vi "Logging Message Loop.vi"(8 "error in (no error)":errorcluster, 10 "Data Queue":refnum<queue>, 11 "Message Queues":T1) -> (0 "error out":errorcluster)   [LabVIEW 2017, in "Logging.lvlib"]
doc: "The message loop subVI to handle messages pertaining to logging data."
uses:
  Logging.lvlib
  support/Message Queue/All Message Queues.ctl
  support/Message Queue/Message Cluster.ctl
  Logging Configuration.ctl
  Logging State.ctl
  support/Message Queue/Enqueue Message (Single).vi
  <vilib>/Utility/error.llb/Error Cluster From Error Code.vi
  <vilib>/ErrorRing/Error Ring.xnode
  support/Message Queue/Message Queue.lvlib
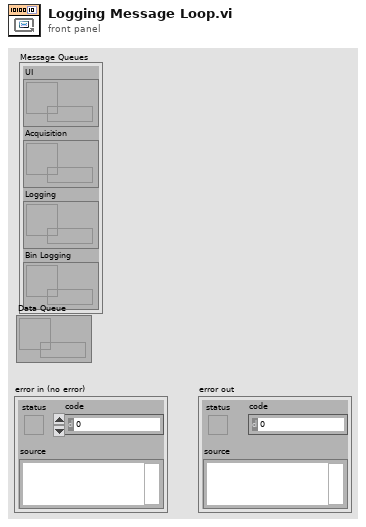
[diagram p1: front panel]
types:
  T1 = typedef "Message Queue.lvlib/All Message Queues.ctl" = cluster{"UI":refnum<queue>, "Acquisition":refnum<queue>, "Logging":refnum<queue>, "Bin Logging":refnum<queue>}
  T2 = typedef "Logging.lvlib/Logging Configuration.ctl" = cluster{"Log File Base Path":path, "TDMS File Reference":refnum<k34>, "Log File Offsite Path":path, "Offsite storage?":bool, "Project code":string, "Max writing time to a file [min]":dbl, "Bin File Reference":refnum<file>}
  T3 = typedef "Logging.lvlib/Logging State.ctl" = enum16{"Idle", "Logging"}
  T4 = enum16{"open", "open or create", "create or replace", "create", "open (read-only)"}
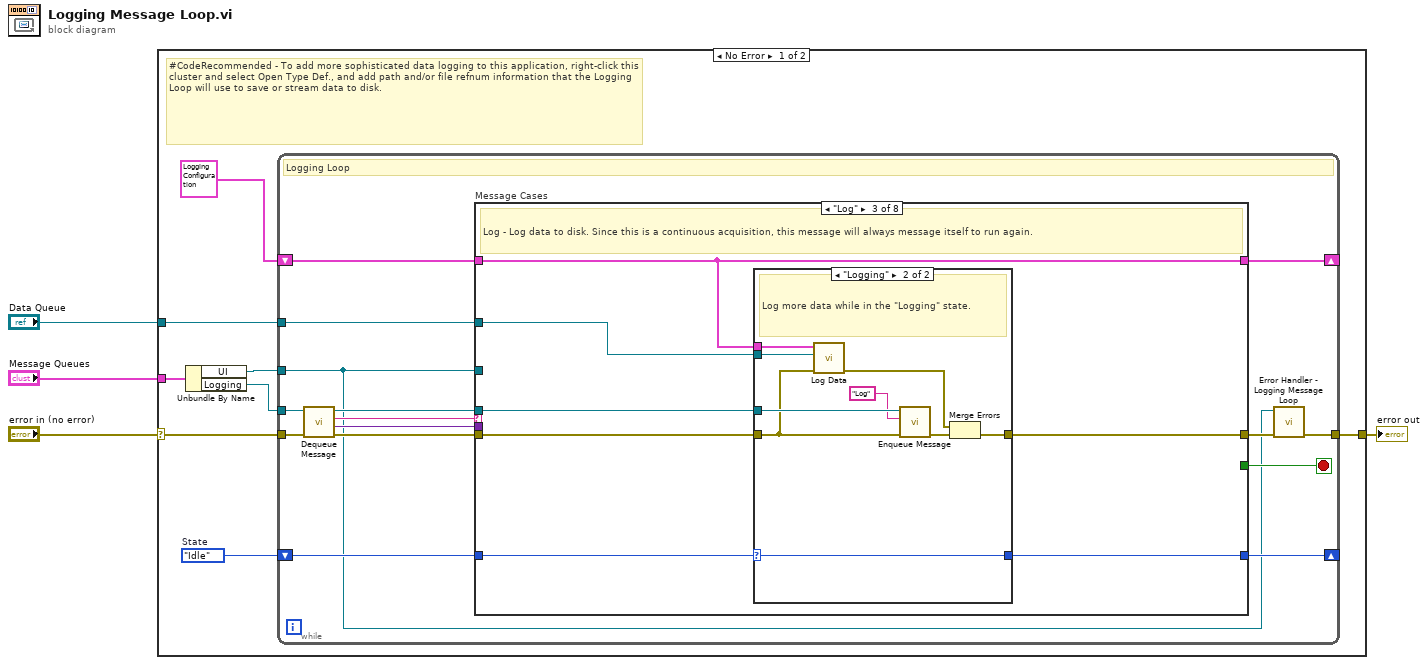
[diagram p0: block diagram]
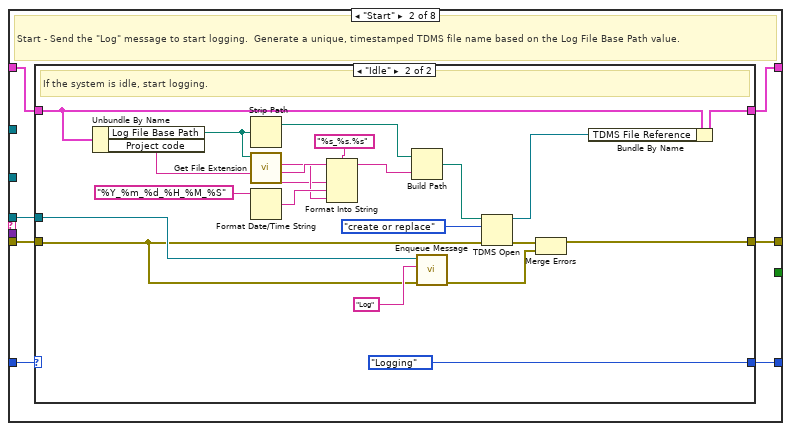
[diagram p3: hidden frame]
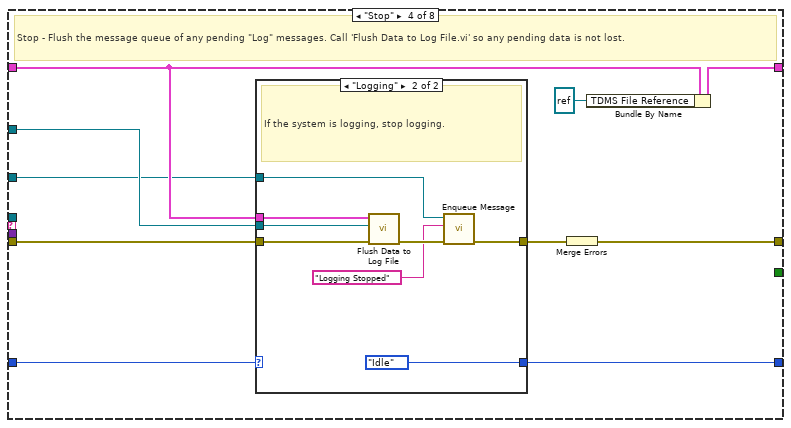
[diagram p6: hidden frame]
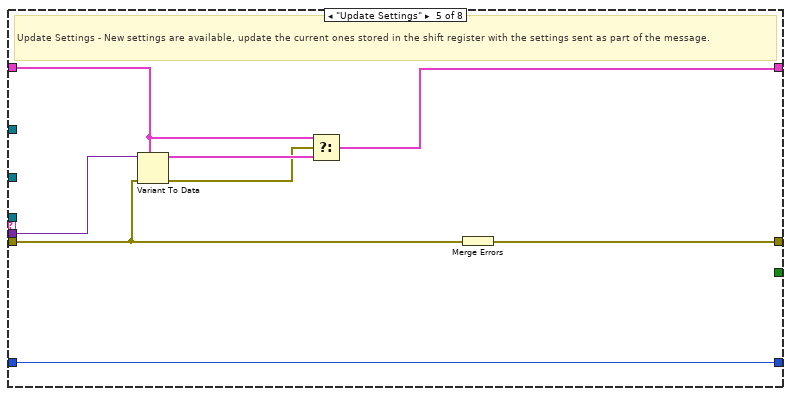
[diagram p8: hidden frame]
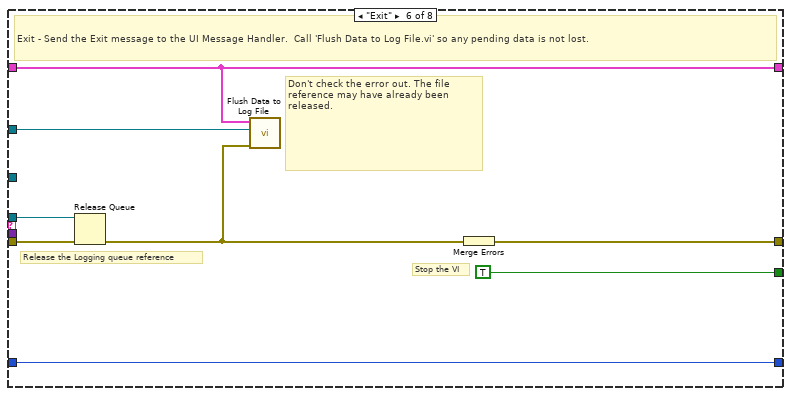
[diagram p9: hidden frame]
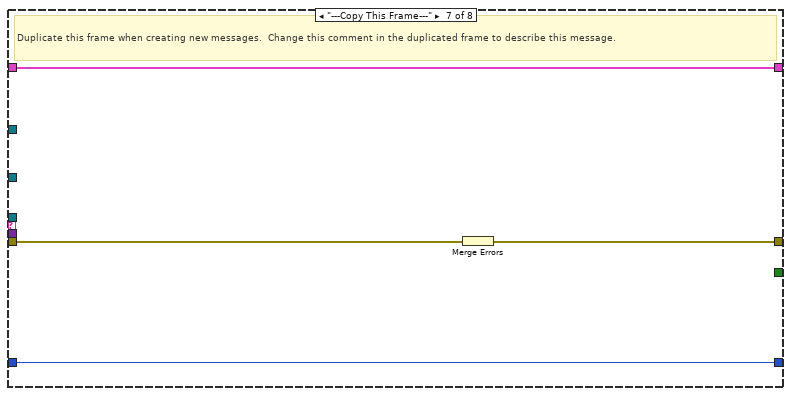
[diagram p10: hidden frame]
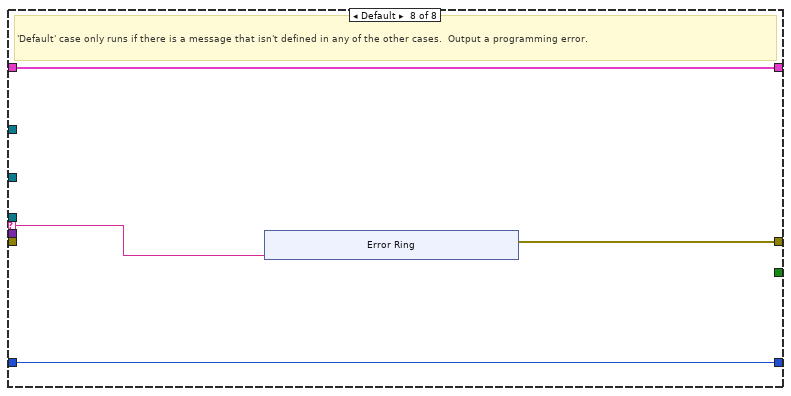
[diagram p11: hidden frame]
diagram:
  n1 = case shown="No Error" "error in (no error)" {
    selector: "error in (no error)" -> [w8 w131]
    tunnel: "Message Queues" -> [w12 _]
    tunnel: [w10 w131] -> w3
    tunnel: "Data Queue" -> [w7 _]
    frame No Error {
      w5 = Logging_State."Idle"  # State
      # "#CodeRecommended - To add more sophisticated data logging to this application, right-click this cluster and select Open Type Def., and add path and/or file refnum information that the Logging Loop will use to save or stream data to disk."
      n2 = Unbundle By Name(w12) -> ("UI"=w6:refnum<queue>, "Logging"=w11:refnum<queue>)
      n3 = while {
        tunnel: w11 -> [w19]
        shift-right: [w26] -> _
        shift-left: T2 {"Log File Base Path"=path "", "TDMS File Reference"=refnum, "Log File Offsite Path"=path "", "Offsite storage?"=FALSE, "Project code"="", "Max writing time to a file [min]"=0.0, "Bin File Reference"=refnum} ("Logging Configuration") -> [w27]
        tunnel: w6 -> [w13]
        tunnel: w7 -> [w18]
        shift-right: [w16] -> _
        shift-left: w5 -> [w17]
        tunnel: w8 -> [w24]
        tunnel: [w15] -> w10
        stop <- w25 stop-if-true
        # "Logging Loop"
        n4 = call "Dequeue Message.vi"("error in (no error)"=w24, "Message Queue"=w19) -> ("error out"=w23:errorcluster, "Message Data"=w21:variant, "Message"=w22:string, "dup Message Queue"=w20:refnum<queue>)  [unwired: 6 in]
        n5 = case "Message Cases" shown="\"Log\"" w22 {
          selector: w22 -> [_ _ _ _ _ _ _ w120]
          tunnel: w20 -> [_ w36 w67 _ _ w112 _ _]
          tunnel: w23 -> [w29 w35 w65 w83 w101 w113 w119 _]
          tunnel: [w29 w37 w68 w89 w107 w114 w117 w121] -> w14
          tunnel: w27 -> [w30 w34 w64 w84 w105 w110 w118 w123]
          tunnel: [w30 w33 w64 w87 w102 w110 w118 w123] -> w26
          tunnel: [_ _ _ _ _ TRUE _ _] -> w25
          tunnel: w21 -> [_ _ _ _ w106 _ _ _]
          tunnel: w13 -> [_ _ _ w80 _ _ _ _]
          tunnel: w18 -> [_ _ w66 w85 _ w109 _ _]
          tunnel: w17 -> [w28 w32 w63 w82 w100 w108 w116 w122]
          tunnel: [w28 w31 w62 w81 w100 w108 w116 w122] -> w16
          frame "Initialize" {
            # "Initialize - gets called when first launched. Currently a no-op."
          }
          frame "Start" {
            # "Start - Send the \"Log\" message to start logging.  Generate a unique, timestamped TDMS file name based on the Log File Base Path value."
            n6 = case shown="\"Idle\"" w32 {
              selector: w32 -> [w39 _]
              tunnel: [w38 w43] -> w37
              tunnel: w36 -> [_ w44]
              tunnel: w35 -> [w38 w42]
              tunnel: w34 -> [w40 w45]
              tunnel: [w40 w47] -> w33
              tunnel: [w39 Logging_State."Logging" ("State")] -> w31
              frame "Logging" {
                # "The system is already logging. Ignore the \"Start\" message."
              }
              frame "Idle" {
                # "If the system is idle, start logging."
                n7 = Unbundle By Name(w45) -> ("Log File Base Path"=w60:path, "Project code"=w41:string)
                n8 = Strip Path(path=w60) -> (stripped path=w57:path)  [unwired: 1 out]
                n9 = call <vilib>:"Get File Extension.vi"("file"=w60) -> ("filename without extension"=w58:string, "lowercase file extension"=w54:string)  [unwired: 6 in, 3 out]
                n10 = Format Date/Time String(time format string (%c)="%Y_%m_%d_%H_%M_%S") -> (date/time string=w55:string)  [unwired: 2 in]
                n11 = Format Into String(format string="%s_%s.%s", initial string=w58, w41, w55, w54) -> (resulting string=w53:string)  [unwired: 1 in, 1 out]
                n12 = Build Path(base path=w57, name or relative path=w53) -> (appended path=w52:path)
                n13 = call-poly "Enqueue Message.vi"("error in (no error)"=w42, "Message"="Log", "Message Queue"=w44) -> ("error out"=w50:errorcluster)  [unwired: 7 in, 1 out]
                n14 = TDMS Open(8:w42, 10:T4."create or replace" ("operation (0:open)"), 11:w52) -> (0:w51:errorcluster, 3:w48:refnum<k34>)  [unwired: 4 in]
                n15 = Merge Errors(w51, w50) -> (w43:errorcluster)
                n16 = Bundle By Name(cluster=w45, "TDMS File Reference"=w48) -> (w47:T2)
              }
            }
          }
          frame "Log" {
            # "Log - Log data to disk. Since this is a continuous acquisition, this message will always message itself to run again."
            n17 = case shown="\"Logging\"" w63 {
              selector: w63 -> [w70 w72]
              tunnel: [w69 w79] -> w68
              tunnel: w67 -> [_ w77]
              tunnel: w66 -> [_ w76]
              tunnel: w65 -> [w69 w71]
              tunnel: w64 -> [_ w73]
              tunnel: [w70 w72] -> w62
              frame "Idle" {
                # "Ignore \"Log\" messages when the logging is idle."
              }
              frame "Logging" {
                # "Log more data while in the \"Logging\" state."
                n18 = call "Log Data.vi"("error in (no error)"=w71, "Data Queue"=w76, "Logging Configuration"=w73) -> ("error out"=w75:errorcluster)  [unwired: 8 in]
                n19 = call-poly "Enqueue Message.vi"("error in (no error)"=w71, "Message"="Log", "Message Queue"=w77) -> ("error out"=w78:errorcluster)  [unwired: 7 in, 1 out]
                n20 = Merge Errors(w75, w78) -> (w79:errorcluster)
              }
            }
          }
          frame "Stop" {
            # "Stop - Flush the message queue of any pending \"Log\" messages. Call 'Flush Data to Log File.vi' so any pending data is not lost."
            n21 = case shown="\"Logging\"" w82 {
              selector: w82 -> [w90 _]
              tunnel: [w91 w94] -> w88
              tunnel: w85 -> [_ w98]
              tunnel: w84 -> [_ w97]
              tunnel: w83 -> [w91 w96]
              tunnel: [w90 Logging_State."Idle" ("State")] -> w81
              tunnel: w80 -> [_ w93]
              frame "Idle" {
                # "The system is already idle. Ignore the \"Stop\" message."
              }
              frame "Logging" {
                # "If the system is logging, stop logging."
                n22 = call "Flush Data to Log File.vi"("error in (no error)"=w96, "Data Queue"=w98, "Logging Configuration"=w97) -> ("error out"=w99:errorcluster)  [unwired: 8 in]
                n23 = call-poly "Enqueue Message.vi"("error in (no error)"=w99, "Message"="Logging Stopped", "Message Queue"=w93) -> ("error out"=w94:errorcluster)  [unwired: 7 in, 1 out]
              }
            }
            n24 = Merge Errors(w88) -> (w89:errorcluster)
            n25 = Bundle By Name(cluster=w84, "TDMS File Reference"=refnum<k34> refnum) -> (w87:T2)
          }
          frame "Update Settings" {
            # "Update Settings - New settings are available, update the current ones stored in the shift register with the settings sent as part of the message."
            n26 = Variant To Data(error in=w101, type=w105, Variant=w106) -> (data=w104:T2, error out=w103:errorcluster)
            n27 = Select(t=w105, s=w103, f=w104) -> (s? t:f=w102:T2)
            n28 = Merge Errors(w101) -> (w107:errorcluster)
          }
          frame "Exit" {
            # "Don't check the error out. The file reference may have already been released."
            # "Release the Logging queue reference"
            # "Stop the VI"
            # "Exit - Send the Exit message to the UI Message Handler.  Call 'Flush Data to Log File.vi' so any pending data is not lost."
            n29 = Release Queue(queue=w112, error in (no error)=w113) -> (error out=w111:errorcluster)  [unwired: 1 in, 2 out]
            n30 = call "Flush Data to Log File.vi"("error in (no error)"=w111, "Data Queue"=w109, "Logging Configuration"=w110) -> ()  [unwired: 8 in, 1 out]
            n31 = Merge Errors(w111) -> (w114:errorcluster)
          }
          frame "---Copy This Frame---" {
            # "Duplicate this frame when creating new messages.  Change this comment in the duplicated frame to describe this message."
            n32 = Merge Errors(w119) -> (w117:errorcluster)
          }
          frame Default {
            # "'Default' case only runs if there is a message that isn't defined in any of the other cases.  Output a programming error."
            n33 = xnode "Error Ring"("parameter 0"=w120) -> ("error out"=w121:errorcluster)
          }
        }
        n34 = call "Error Handler - Logging Message Loop.vi"("error in (no error)"=w14, "Message Queue"=w13) -> ("dup error in"=w15:errorcluster)  [unwired: 8 in, 1 out]
      }
    }
    frame Error {
    }
  }
  "error out" <- w3
